vi "LAUNCHER.vi"   [LabVIEW 2020]
uses:
  UI/UI.lvclass
  C:/Program Files (x86)/National Instruments/LabVIEW 2020/vi.lib/ActorFramework/Actor/Actor.lvclass
  <vilib>/ActorFramework/Actor/Actor.lvclass
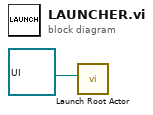
[diagram p0: block diagram]
diagram:
  n1 = call <vilib>:"Launch Root Actor.vi"("Actor"=refnum<class "UI.lvclass"> refnum ("UI.lvlib:UI.lvclass")) -> ()  [unwired: 9 in, 2 out]
